vi "makeSampleFromAtlas.vi"(6 "Centre":i32[](array[numeric]), 8 "Image Properties":T1, 9 "slice":u32, 10 "tiff pointer":i64, 11 "Angle":dbl) -> (3 "Forward Projection":sgl[](array[numeric]))   [LabVIEW 2013]
uses:
  tags_cluster.ctl
  imagereconstruction/x64/Debug/labviewdll.dll
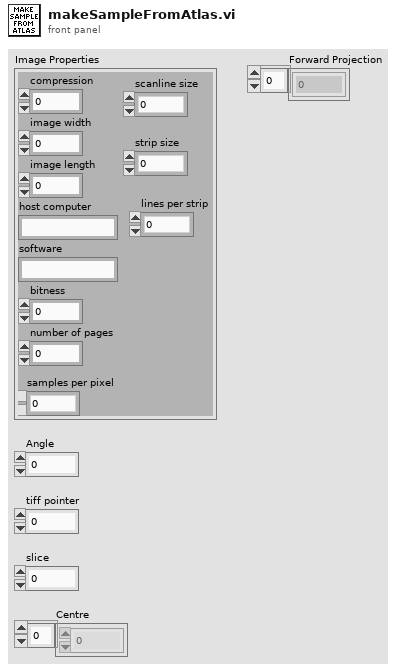
[diagram p1: front panel]
types:
  T1 = typedef "tags_cluster.ctl" = cluster{"compression":i32, "image width":i32, "image length":i32, "host computer":string, "software":string, "bitness":i32, "number of pages":i32, "samples per pixel":i32, "scanline size":i32, "strip size":i32, "lines per strip":i32}
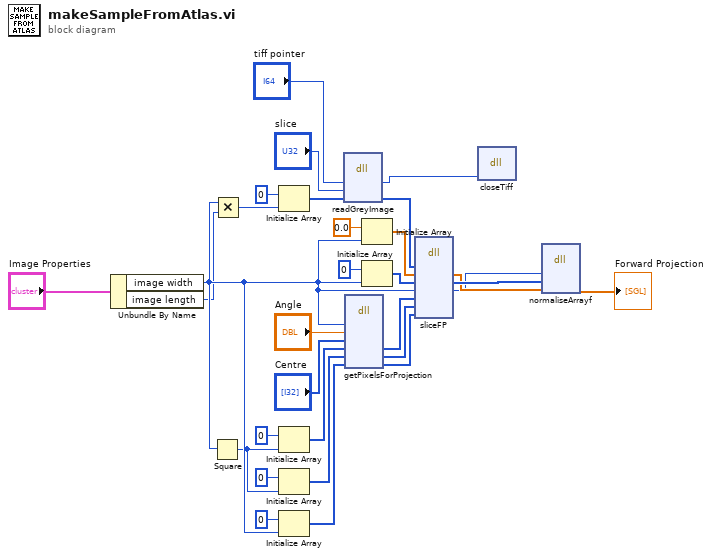
[diagram p0: block diagram]
diagram:
  n1 = Unbundle By Name("Image Properties") -> ("image width"=w24:i32, "image length"=w5:i32)
  n2 = Square(x=w24) -> (x^2=w16:i32)
  n3 = Multiply(x=w24, y=w5) -> (x*y=w6:i32)
  n4 = Initialize Array(u8 0 ("element"), w6) -> (w8:u8[])
  n5 = Initialize Array(0 ("element"), w16) -> (w14:i32[])
  n6 = Initialize Array(0 ("element"), w16) -> (w17:i32[])
  n7 = Initialize Array(0 ("element"), w24) -> (w12:i32[])
  n8 = dll-call lib="D:/work/uni/FYP/reconrepo/imagereconstruction/x64/Debug/labviewdll.dll" fn="readGreyImage"("tiff"="tiff pointer", "directory"="slice", "buffer"=w8) -> ("tiff"=w1:i64, "buffer"=w18:u8[])  [unwired: 5 in, 2 out]
  n9 = dll-call lib="D:/work/uni/FYP/reconrepo/imagereconstruction/x64/Debug/labviewdll.dll" fn="getPixelsForProjection"("w"=w24, "angle"="Angle", "centre"="Centre", "normalisation"=w14, "pixels"=w17, "count"=w12) -> ("normalisation"=w21:i32[], "pixels"=w20:i32[], "count"=w19:i32[])  [unwired: 7 in, 2 out]
  n10 = Initialize Array(sgl 0.0 ("element"), w24) -> (w25:sgl[])
  n11 = Initialize Array(0 ("element"), w24) -> (w26:i32[])
  n12 = dll-call lib="D:/work/uni/FYP/reconrepo/imagereconstruction/x64/Debug/labviewdll.dll" fn="sliceFP"("object"=w18, "projection"=w25, "normalisation"=w26, "w"=w24, "rayNormalisation"=w21, "pixels"=w20, "count"=w19) -> ("projection"=w28:sgl[], "normalisation"=w29:i32[], "w"=w27:i32)  [unwired: 8 in, 2 out]
  n13 = dll-call lib="D:/work/uni/FYP/reconrepo/imagereconstruction/x64/Debug/labviewdll.dll" fn="closeTiff"("tiff"=w1) -> ()  [unwired: 5 in, 2 out]
  n14 = dll-call lib="D:/work/uni/FYP/reconrepo/imagereconstruction/x64/Debug/labviewdll.dll" fn="normaliseArrayf"("length"=w27, "normalisation"=w29, "normalisedArray"=w28) -> ("normalisedArray"=→"Forward Projection":sgl[])  [unwired: 6 in, 2 out]
